vi "DateToBDD.vi"(11 "in":string="03/04/2023_08:40:52") -> (3 "out":string)   [LabVIEW 2020]
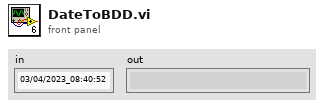
[diagram p1: front panel]
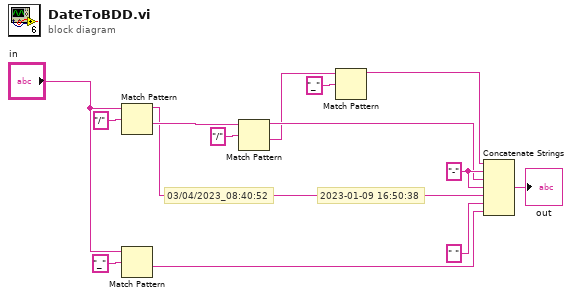
[diagram p0: block diagram]
diagram:
  w10 = "-" ("string")
  # "03/04/2023_08:40:52"
  # "2023-01-09 16:50:38"
  n1 = Match Pattern(string="in", regular expression="/") -> (before substring=w6:string, after substring=w11:string)  [unwired: 1 in, 2 out]
  n2 = Match Pattern(string="in", regular expression="_") -> (after substring=w7:string)  [unwired: 1 in, 3 out]
  n3 = Match Pattern(string=w11, regular expression="/") -> (before substring=w5:string, after substring=w2:string)  [unwired: 1 in, 2 out]
  n4 = Match Pattern(string=w2, regular expression="_") -> (before substring=w1:string)  [unwired: 1 in, 3 out]
  n5 = Concatenate Strings(w1, w10, w5, w10, w6, " " ("string"), w7) -> (→"out":string)
